vi "Data_In_assessment.vi"(3 "Array":dbl[](array[numeric])) -> (0 "Message Form":T2, 1 "Types of Data":T1)   [LabVIEW 2016]
uses:
  Message_info.ctl
  Type_of_message_to_MCU.ctl
  <vilib>/Utility/file.llb/Read Delimited Spreadsheet (DBL).vi
panel:
  out "all rows":dbl[][](array[numeric])
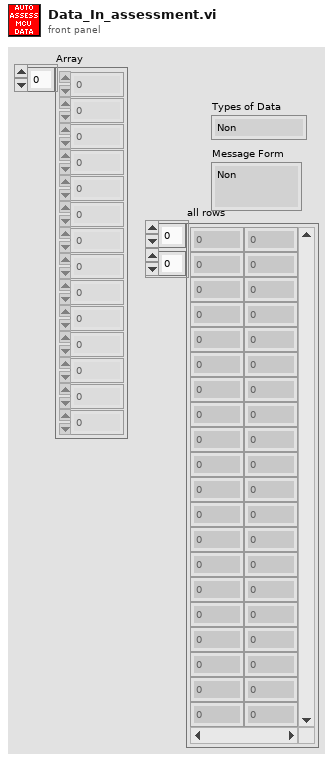
[diagram p1: front panel]
types:
  T1 = typedef "Type_of_message_to_MCU.ctl" = enum16{"Non", "Alarm", "Error", "Time and Date", "Status", "Request"}
  T2 = typedef "Message_info.ctl" = enum16{"Non", "Earthquake", "Fire", "Lost Power", "New", "Restarted"}
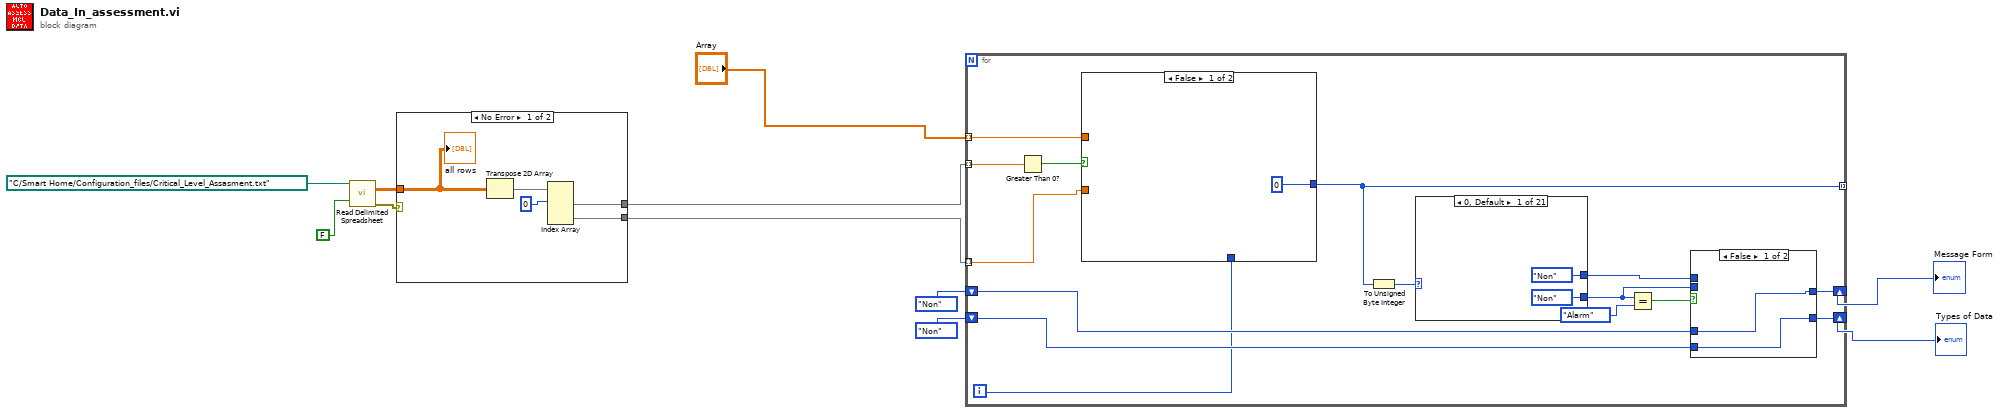
[diagram p0: block diagram]
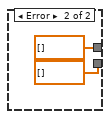
[diagram p2: hidden frame]
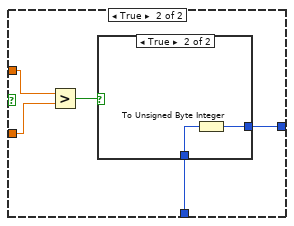
[diagram p3: hidden frame]
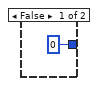
[diagram p4: hidden frame]
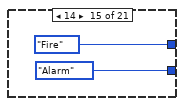
[diagram p19: hidden frame]
diagram:
  n1 = call-poly <vilib>:"Read Delimited Spreadsheet.vi"("file path (dialog if empty)"=path "C:/Smart Home/Configuration_files/Critical_Level_Assasment.txt", "transpose? (F)"=FALSE) -> ("all rows"=w5:dbl[][], "error out"=w1:errorcluster)  [unwired: 8 in, 4 out]
  n2 = case shown="No Error" w1 {
    tunnel: w5 -> [w16 _]
    tunnel: [w14 dbl[] []] -> w4
    tunnel: [w13 dbl[] []] -> w3
    frame No Error {
      n3 = Transpose 2D Array(2D array=w16) -> (transposed array=w12:dbl[][])
      n4 = Index Array(array=w12, index (row) #1=0 ("index (row)")) -> (element #1=w14:dbl[], element #2=w13:dbl[])  [unwired: 3 in]
      "all rows" <- w16
    }
    frame Error {
    }
  }
  n5 = for {
    tunnel: w3 -> [w20] mode=indexing
    tunnel: "Array" -> [w21] mode=indexing
    tunnel: [w33] -> _ mode=indexing
    shift-right: [w27] -> w8
    shift-left: Message_info."Non" ("Message Form") -> [w25]
    shift-right: [w26] -> w7
    shift-left: Type_of_message_to_MCU."Non" ("Types of Data") -> [w24]
    tunnel: w4 -> [w23] mode=indexing
    i -> [w19]
    n6 = Greater Than 0?(x=w23) -> (x > 0?=w22:bool)
    n7 = case shown="False" w22 {
      tunnel: [u8 0 w35] -> w33
      tunnel: w21 -> [_ w38]
      tunnel: w20 -> [_ w37]
      tunnel: w19 -> [_ w36]
      frame False {
      }
      frame True {
        n8 = Greater?(x=w38, y=w37) -> (0:w39:bool)
        n9 = case shown="True" w39 {
          tunnel: [u8 0 w41] -> w35
          tunnel: w36 -> [_ w42]
          frame False {
          }
          frame True {
            n10 = To Unsigned Byte Integer(number=w42) -> (unsigned 8bit integer=w41:u8)
          }
        }
      }
    }
    n11 = To Unsigned Byte Integer(number=w33) -> (unsigned 8bit integer=w32:u8)
    n12 = case shown="0, Default" w32 {
      tunnel: [Message_info."Non" ("Message Form") _ _ _ _ _ _ _ _ _ _ _ _ _ Message_info."Fire" ("Message Form") _ _ _ Message_info."Fire" ("Message Form") _ _] -> w28
      tunnel: [Type_of_message_to_MCU."Non" ("Types of Data") _ _ _ _ _ _ _ _ _ _ _ _ _ Type_of_message_to_MCU."Alarm" ("Types of Data") _ _ _ Type_of_message_to_MCU."Alarm" ("Types of Data") _ _] -> w29
      frame 0, Default {
      }
      frame 1 {
      }
      frame 2 {
      }
      frame 3 {
      }
      frame 4 {
      }
      frame 5 {
      }
      frame 6 {
      }
      frame 7 {
      }
      frame 8 {
      }
      frame 9 {
      }
      frame 10 {
      }
      frame 11 {
      }
      frame 12 {
      }
      frame 13 {
      }
      frame 14 {
      }
      frame 15 {
      }
      frame 16 {
      }
      frame 17 {
      }
      frame 18 {
      }
      frame 19 {
      }
      frame 20 {
      }
    }
    n13 = Equal?(x=w29, y=Type_of_message_to_MCU."Alarm" ("Types of Data")) -> (x = y?=w30:bool)
    n14 = case shown="False" w30 {
      tunnel: w29 -> [_ w45]
      tunnel: w28 -> [_ w46]
      tunnel: [w44 w46] -> w27
      tunnel: [w43 w45] -> w26
      tunnel: w25 -> [w44 _]
      tunnel: w24 -> [w43 _]
      frame False {
      }
      frame True {
      }
    }
  }
  "Message Form" <- w8
  "Types of Data" <- w7
